vi "SV Limit Testing for Monitoring (waveform) (SGL).vi"(7 "reset":bool, 9 "lower limit":sgl=-inf format="%.2f", 10 "upper limit":sgl=inf format="%.2f", 11 "signal in":waveform(sgl)) -> (1 "lower limit clearance":sgl format="%.6f", 2 "upper limit clearance":sgl format="%.6f", 3 "test passed?":bool, 5 "timestamp":timestamp format="%<%.6X\n%x>T")   [LabVIEW 2017]
doc: "Performs limit testing on waveforms, spectra, XY data, identified peaks, or scalar measurements. You can wire <B>output values</B> to a graph to view the limits, signal, and failures. Wire data to the<B> signal in</B> input to determine the polymorphic instance to use or manually select the instance."
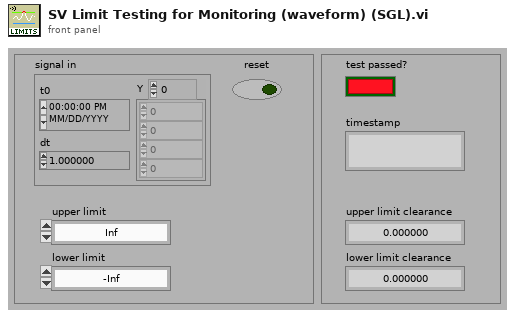
[diagram p1: front panel]
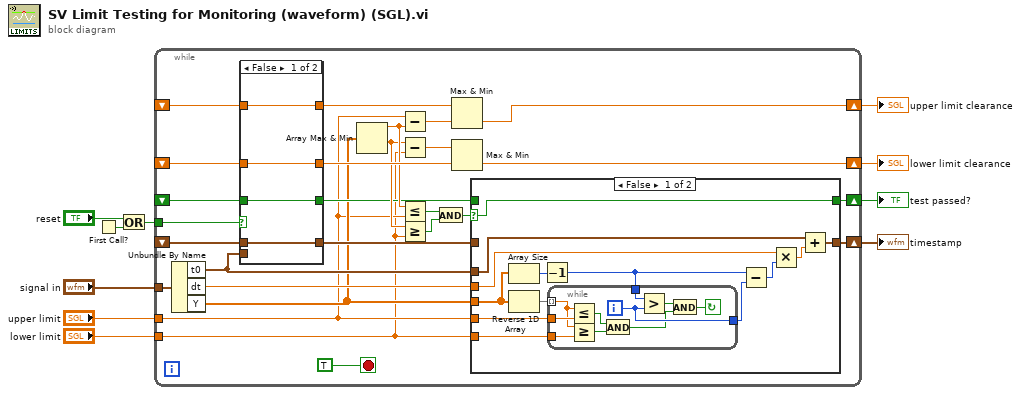
[diagram p0: block diagram]
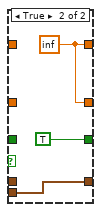
[diagram p3: hidden frame]
diagram:
  n1 = First Call?() -> (First Call?: T/F=w2:bool)
  n2 = Or(x="reset", y=w2) -> (x .or. y?=w3:bool)
  n3 = while {
    tunnel: "signal in" -> [w37]
    tunnel: "upper limit" -> [w14]
    tunnel: "lower limit" -> [w13]
    shift-right: [w36] -> w7
    shift-left: _ -> [w33]
    shift-right: [w35] -> w6
    shift-left: _ -> [w31]
    shift-right: [w12] -> w5
    shift-left: _ -> [w29]
    shift-right: [w11] -> w1
    shift-left: _ -> [w28]
    tunnel: w3 -> [w34]
    stop <- TRUE stop-if-true
    n4 = Unbundle By Name(w37) -> ("t0"=w17:timestamp, "dt"=w16:dbl, "Y"=w15:sgl[])
    n5 = case shown="False" w34 {
      tunnel: w33 -> [w66 _]
      tunnel: [w66 w67] -> w32
      tunnel: w31 -> [w65 _]
      tunnel: [w65 w67] -> w30
      tunnel: w29 -> [w64 _]
      tunnel: [w64 TRUE] -> w20
      tunnel: w28 -> [w63 _]
      tunnel: [w63 w69] -> w18
      tunnel: w17 -> [_ w69]
      frame False {
      }
      frame True {
        w67 = sgl inf
      }
    }
    n6 = Array Max & Min(array=w15) -> (max value=w22:sgl, min value=w21:sgl)  [unwired: 2 out]
    n7 = Subtract(x=w14, y=w22) -> (x-y=w24:sgl)
    n8 = Subtract(x=w21, y=w13) -> (x-y=w23:sgl)
    n9 = Less Or Equal?(x=w22, y=w14) -> (x <= y?=w26:bool)
    n10 = Greater Or Equal?(x=w21, y=w13) -> (x >= y?=w25:bool)
    n11 = And(x=w26, y=w25) -> (x .and. y?=w19:bool)
    n12 = Max & Min(x=w32, y=w24) -> (min(x,y)=w36:sgl)  [unwired: 1 out]
    n13 = Max & Min(x=w23, y=w30) -> (min(x,y)=w35:sgl)  [unwired: 1 out]
    n14 = case shown="False" w19 {
      selector: w19 -> [w47 _]
      tunnel: w18 -> [_ w62]
      tunnel: [w49 w62] -> w11
      tunnel: w17 -> [w50 _]
      tunnel: w16 -> [w46 _]
      tunnel: w20 -> [_ w61]
      tunnel: [w47 w61] -> w12
      tunnel: w15 -> [w38 _]
      tunnel: w14 -> [w45 _]
      tunnel: w13 -> [w44 _]
      frame False {
        n15 = Array Size(array=w38) -> (size(s)=w42:i32)
        n16 = Reverse 1D Array(array=w38) -> (reversed array=w43:sgl[])
        n17 = Decrement(x=w42) -> (x-1=w41:i32)
        n18 = while {
          tunnel: [w54] -> w40
          tunnel: w45 -> [w58]
          tunnel: w44 -> [w57]
          tunnel: w43 -> [w56] mode=indexing
          tunnel: w41 -> [w55]
          i -> [w54]
          stop <- w51 continue-if-true
          n19 = Less Or Equal?(x=w56, y=w58) -> (x <= y?=w60:bool)
          n20 = Greater Or Equal?(x=w56, y=w57) -> (x >= y?=w59:bool)
          n21 = And(x=w60, y=w59) -> (x .and. y?=w52:bool)
          n22 = Greater?(x=w55, y=w54) -> (0:w53:bool)
          n23 = And(x=w53, y=w52) -> (x .and. y?=w51:bool)
        }
        n24 = Subtract(x=w41, y=w40) -> (x-y=w39:i32)
        n25 = Multiply(x=w46, y=w39) -> (x*y=w48:dbl)
        n26 = Add(x=w50, y=w48) -> (x+y=w49:timestamp)
      }
      frame True {
      }
    }
  }
  "test passed?" <- w5
  "upper limit clearance" <- w7
  "lower limit clearance" <- w6
  "timestamp" <- w1
